vi "ActiView806-Lores.vi"() -> ()   [LabVIEW 2020] (continued)
          # "Average Cluster"
          # "Tab Control"
          # "Last Call"
          # "Stop next call"
          # "Update Avg"
          # "Average Cluster"
          # "Average Total"
          # "Noise Total"
          # "Decimation Factor"
          # "Ana Filter Reset"
          # "Ana Filter Reset"
          # "Ana Channel Selection"
          # "Charts/Graphs"
          # "Ana Channel Selection"
          # "Acquisition Error"
          # "Second Half"
          # "Aux Channel Selection"
          # "Aux Channel Selection"
          # "Aux DC Reset"
          # "Aux DC Reset"
          # "Save Index"
          # "Bip Channel Selection"
          # "Bip Channel Selection"
          # "Sample Rate"
          # "Mon Channel selection"
          # "Mon Ref Selection"
          # "Mon Channel selection"
          # "Mon Ref Selection"
          # "Bip Filter Reset"
          # "Bip Filter Reset"
          # "Mon Filter Reset"
          # "Mon Filter Reset"
          # "Max/Min Display Blocksize"
          # "Popup Change"
          # "Popups Change"
          # "Max/Min Display Blocksize"
          # "Screen Reset"
          # "Current File in Byte"
          # "Header Lenght in Byte"
          # "Header Lenght in Byte"
          # "Current File in Byte"
          # "Screen Reset"
          # "Sync Error Cluster"
          # "Sync Error Cluster"
          # "Display/Save data until an error occurs,\nor Stop or Start-File button is pressed"
          # "No Incoming Data"
          # "Buffer Pointer"
          # "Buffer pointer"
          # "Speed/Save Cluster"
          # "Start Saving"
          # "New Total Buffered"
          # "Save Array"
          # "Diplay Blocksize"
          # "Display Index"
          # "Display Blocksize"
          # "New Total Displayed"
          # "Total ADC Samples/s"
          # "New Total Buffered"
          # "Buffer Size in I32"
          # "Old Total Displayed"
          # "New Total Buffered"
          # "Display Index"
          # "Old total buffered"
          n1262 = property class="VI"() -> ("Front Panel Window:Is Frontmost"=w2860:bool)  [unwired: 2 in, 2 out]
          n1263 = global write "StopThreads.glb" "StopThreads"(w2775) -> ()
          n1264 = Wait (ms)(milliseconds to wait=u32 0) -> ()  [unwired: 1 out]
          n1265 = call-poly <vilib>:"Acquire Input Data.vi"("device ID"=w2889, "error in (no error)"=w2888) -> ("device ID"=w2884:refnum<k1>, "keys pressed"=w2864:T29, "error out"=w2885:errorcluster)  [unwired: 15 out]
          n1266 = Less Or Equal?(x=w2910, y=w2905) -> (x <= y?=w2916:bool)
          n1267 = Select(t=w2910, s=w2916, f=w2905) -> (s? t:f=w2911:i64)
          n1268 = call "AVTCP-Pause FGV.vi"() -> ("Value out"=w2757:bool)  [unwired: 7 in]
          n1269 = Greater Or Equal?(x=w2842, y="RecTimeLimit") -> (x >= y?=w2810:bool)
          n1270 = Multiply(x=w2909, y="FileLimit") -> (x*y=w2813:i64)
          n1271 = global read "TCPidentification.glb" "TCP cluster"() -> (w2829:T9)
          n1272 = Quotient & Remainder(x=w2911, y=w2904) -> (floor(x/y)=w2914:i64)  [unwired: 1 out]
          n1273 = property on="MonFree" class="LstBox (strict)"() -> ("Key Focus"=w2791:bool)  [unwired: 2 in, 2 out]
          n1274 = property on="RefFree" class="LstBox (strict)"() -> ("Key Focus"=w2790:bool)  [unwired: 2 in, 2 out]
          n1275 = property on="BipFree" class="LstBox (strict)"() -> ("Key Focus"=w2789:bool)  [unwired: 2 in, 2 out]
          n1276 = property on="AnaFree" class="LstBox (strict)"() -> ("Key Focus"=w2788:bool)  [unwired: 2 in, 2 out]
          n1277 = property on="AnaOffset" class="Ring (strict)"() -> ("Key Focus"=w2786:bool)  [unwired: 2 in, 2 out]
          n1278 = Unbundle By Name(w2875) -> ("ElecGain"=w2876:i8)
          n1279 = Bundle(w2905, w2904) -> (w2805:cluster{i64, i64})  [unwired: 1 out]
          n1280 = Unbundle By Name(w2922) -> ("Valid Sweeps"=w2785:i32, "Rejected Sweeps"=w2783:i32)
          n1281 = And(x=w2757, y="Pause Saving") -> (x .and. y?=w2756:bool)
          n1282 = Select(t=T5."Disabled and Grayed Out" ("Disabled"), s="Averaging", f=T5."Enabled" ("Disabled")) -> (s? t:f=w2779:T5)
          n1283 = Less Or Equal To 0?(x=w2914) -> (x <= 0?=w2915:bool)
          n1284 = local write "Pause Saving"(w2756) -> ()
          n1285 = Select(t=i64 1, s=w2915, f=w2914) -> (s? t:f=w2912:i64)
          n1286 = Compound Arithmetic op=OR(w2791, w2790, w2789, w2788, w2786) -> (w2787:bool)
          n1287 = Unbundle By Name(w2829) -> ("connection ID"=w2824:refnum<k5>, "remote address"=→"Remote Address":string, "remote port"=w2827:u16)
          "Receive Remote Port" <- w2827
          n1288 = Unbundle By Name(w2869) -> ("Save Subset"=w2868:i8)
          n1289 = Multiply(x=w2912, y=w2904) -> (x*y=w2892:i64)
          n1290 = local read "Valid Sweeps"() -> (w2784:i32)
          n1291 = property on="AvgTrigSel" class="LstBox (strict)"("Disabled"=w2779) -> ()  [unwired: 2 in, 2 out]
          n1292 = property on="AvgTrigLog" class="Ring (strict)"("Disabled"=w2779) -> ()  [unwired: 2 in, 2 out]
          n1293 = property on="AvgSweep" class="DigNum (strict)"("Disabled"=w2779) -> ()  [unwired: 2 in, 2 out]
          n1294 = Add(x=w2953, y=w2811) -> (x+y=w2896:i64)
          n1295 = property on="MonLPfreq" class="DigNum (strict)"() -> ("Key Focus"=w2859:bool)  [unwired: 2 in, 2 out]
          n1296 = property on="MonHPfreq" class="DigNum (strict)"() -> ("Key Focus"=w2858:bool)  [unwired: 2 in, 2 out]
          n1297 = property on="BipLPfreq" class="DigNum (strict)"() -> ("Key Focus"=w2857:bool)  [unwired: 2 in, 2 out]
          n1298 = property on="BipHPfreq" class="DigNum (strict)"() -> ("Key Focus"=w2856:bool)  [unwired: 2 in, 2 out]
          n1299 = property on="AvgSweep" class="DigNum (strict)"() -> ("Key Focus"=w2855:bool)  [unwired: 2 in, 2 out]
          n1300 = property on="AvgLPfreq" class="DigNum (strict)"() -> ("Key Focus"=w2854:bool)  [unwired: 2 in, 2 out]
          n1301 = property on="AvgHPfreq" class="DigNum (strict)"() -> ("Key Focus"=w2853:bool)  [unwired: 2 in, 2 out]
          n1302 = Equal To 0?(x=w2897) -> (x = 0?=w2895:bool)
          n1303 = Equal?(x=w2868, y=i8 8) -> (x = y?=w2866:bool)
          n1304 = local read "Charts/Graphs"() -> (w2924:T2)
          n1305 = Greater?(x=w2785, y=w2784) -> (0:w2781:bool)
          n1306 = Not Equal To 0?(x=w2827) -> (x != 0?=w2826:bool)
          "TCP Connected" <- w2826
          n1307 = local read "Rejected Sweeps"() -> (w2782:i32)
          n1308 = Not And(1:w2866, 2:w2755) -> (0:w2865:bool)
          n1309 = call "AVTCP-Saving FGV.vi"("Value in"=w2755) -> ()  [unwired: 6 in, 1 out]
          n1310 = call "Act_Pointer.vi"("First Iteration"=w2895, "Handle In"=w2766, "Display Blocksize In"=w2892, "Buffer Size"=w2893, "Old Total Displayed"=w3002, "Old Total Buffered"=w3003) -> ("Data Ready"=w2963:bool, "No Incoming Data"=w2898:bool, "Buffer Pointer"=w2764:i64, "New Total Buffered"=w2899:i64, "Handle Out"=w2765:i64)
          n1311 = Greater?(x=w2896, y=w2813) -> (0:w2809:bool)
          n1312 = property on="MonFreeAvg1" class="LstBox (strict)"("Disabled"=w2779) -> ()  [unwired: 2 in, 2 out]
          n1313 = property on="RefFreeAvg1" class="LstBox (strict)"("Disabled"=w2779) -> ()  [unwired: 2 in, 2 out]
          n1314 = Compound Arithmetic op=OR(w2787, w2859, w2858, w2857, w2856, w2855, w2854, w2853) -> (w2794:bool)
          n1315 = Greater?(x=w2783, y=w2782) -> (0:w2780:bool)
          n1316 = case shown="True" w2755 {
            tunnel: w2756 -> [_ w3024]
            frame False {
            }
            frame True {
              n1317 = property on="Start Saving" class="Bool (strict)"() -> ("Colors [4]"=w3033:cluster{u32, u32}[])  [unwired: 2 in, 2 out]
              n1318 = Select(t="Not Saving" ("f"), s=w3024, f="Saving" ("Boolean Text.Text")) -> (s? t:f=w3036:string)
              n1319 = Select(t=u32 16711680, s=w3024, f=u32 6618880) -> (s? t:f=w3028:u32)
              n1320 = Index Array(array=w3033) -> (element #1=w3027:cluster{u32, u32}, element #2=w3030:cluster{u32, u32})  [unwired: 2 in]
              n1321 = Select(t=u32 16777215, s=w3024, f=u32 0) -> (s? t:f=w3023:u32)
              n1322 = Unbundle(w3030) -> (w3029:u32)  [unwired: 1 out]
              n1323 = Bundle(w3028, w3029) -> (w3031:cluster{u32, u32})  [unwired: 1 out]
              n1324 = Build Array(w3027, w3031) -> (w3032:cluster{u32, u32}[])
              n1325 = property on="Start Saving" class="Bool (strict)"("Boolean Text.Text"=w3036, "Colors [4]"=w3032, "Boolean Text.Text Colors:Text Color"=w3023) -> ()  [unwired: 2 in, 2 out]
            }
          }
          n1326 = Not Equal?(x=w2803, y=w2767) -> (x != y?=w2925:bool)
          n1327 = Greater Or Equal?(x=w2976, y=w2812) -> (x >= y?=w2835:bool)
          n1328 = Equal?(x=w2767, y=w2924) -> (x = y?=w2777:bool)
          n1329 = Or(x=w2781, y=w2780) -> (x .or. y?=w2778:bool)
          n1330 = Exclusive Or(1:w2834, 2:w2835) -> (0:w2833:bool)
          n1331 = Or(x=w2810, y=w2809) -> (x .or. y?=w2808:bool)
          n1332 = property on="MonFreeAvg2" class="LstBox (strict)"("Disabled"=w2779) -> ()  [unwired: 2 in, 2 out]
          n1333 = property on="RefFreeAvg2" class="LstBox (strict)"("Disabled"=w2779) -> ()  [unwired: 2 in, 2 out]
          n1334 = And(x=w2778, y=w2777) -> (x .and. y?=w2776:bool)
          n1335 = And(x=w2925, y=w2777) -> (x .and. y?=w2771:bool)
          n1336 = Not And(1:w2833, 2:w2755) -> (0:w2836:bool)
          n1337 = Not And(1:w2755, 2:w2808) -> (0:w2968:bool)
          n1338 = local write "Start"(TRUE ("Start")) -> ()
          n1339 = Select(t=w3012, s=w2963, f=w3013) -> (s? t:f=w2838:i8)
          n1340 = property on="AvgScale" class="DigNum (strict)"() -> ("Key Focus"=w2852:bool)  [unwired: 2 in, 2 out]
          n1341 = property on="AvgAbsReject" class="DigNum (strict)"() -> ("Key Focus"=w2851:bool)  [unwired: 2 in, 2 out]
          n1342 = property on="AvgRelReject" class="DigNum (strict)"() -> ("Key Focus"=w2850:bool)  [unwired: 2 in, 2 out]
          n1343 = property on="AnaLPfreq" class="DigNum (strict)"() -> ("Key Focus"=w2849:bool)  [unwired: 2 in, 2 out]
          n1344 = property on="AnaHPfreq" class="DigNum (strict)"() -> ("Key Focus"=w2848:bool)  [unwired: 2 in, 2 out]
          n1345 = property on="FileLimit" class="DigNum (strict)"() -> ("Key Focus"=w2847:bool)  [unwired: 2 in, 2 out]
          n1346 = property on="RecTimeLimit" class="DigNum (strict)"() -> ("Key Focus"=w2846:bool)  [unwired: 2 in, 2 out]
          n1347 = Compound Arithmetic op=OR(w2776, w2775, w2771) -> (w2774:bool)
          n1348 = Not Or(1:w2756, 2:w2836) -> (0:→"Write":bool)
          n1349 = property on="AvgLP" class="Bool (strict)"("Disabled"=w2779) -> ()  [unwired: 2 in, 2 out]
          n1350 = property on="AvgLPfreq" class="DigNum (strict)"("Disabled"=w2779) -> ()  [unwired: 2 in, 2 out]
          n1351 = Not And(1:"Averaging", 2:w2774) -> (0:w2773:bool)
          n1352 = Select(t=w2838, s=w2773, f=w2927) -> (s? t:f=w2837:i8)
          n1353 = Select(t=w2837, s=w2836, f=w3011) -> (s? t:f=w2993:i8)
          n1354 = Compound Arithmetic op=OR(w2794, w2852, w2851, w2850, w2849, w2848, w2847, w2846) -> (w2793:bool)
          n1355 = property on="AvgHP" class="Bool (strict)"("Disabled"=w2779) -> ()  [unwired: 2 in, 2 out]
          n1356 = property on="AvgHPfreq" class="DigNum (strict)"("Disabled"=w2779) -> ()  [unwired: 2 in, 2 out]
          n1357 = Select(t=w2993, s=w2968, f=w2997) -> (s? t:f=w2839:i8)
          n1358 = Not(x=w2793) -> (.not. x?=w2792:bool)
          n1359 = And(x=w2860, y=w2792) -> (x .and. y?=w2861:bool)
          n1360 = Select(t=w2864, s=w2861, f=w2862) -> (s? t:f=w2863:T29)
          n1361 = Index Array(array=w2863) -> (element=w2872:T12)  [unwired: 1 in]
          n1362 = Equal?(x=w2872, y=T12."PRIOR (PG UP)") -> (x = y?=w2882:bool)
          n1363 = Equal?(x=w2872, y=T12."UP") -> (x = y?=w2886:bool)
          n1364 = Equal?(x=w2872, y=T12."NEXT") -> (x = y?=w2883:bool)
          n1365 = Equal?(x=w2872, y=T12."DOWN") -> (x = y?=w2887:bool)
          n1366 = Equal?(x=w2872, y=T12."RIGHT") -> (x = y?=w2822:bool)
          n1367 = Equal?(x=w2872, y=T12."LEFT") -> (x = y?=w2870:bool)
          n1368 = Or(x=w2870, y=w2822) -> (x .or. y?=w2821:bool)
          n1369 = case shown="\"Monopolar Display\"" w2803 {
            tunnel: w2887 -> [w3071 w3108 w3125 w3166 _]
            tunnel: w2886 -> [w3073 w3109 w3124 w3165 _]
            tunnel: w2883 -> [w3069 _ w3120 _ _]
            tunnel: w2882 -> [w3070 _ w3121 _ _]
            tunnel: w2881 -> [w3068 _ _ _ _]
            tunnel: w2876 -> [_ _ w3123 _ _]
            tunnel: w2874 -> [_ _ w3122 _ _]
            tunnel: w2865 -> [w3067 _ _ _ _]
            frame "Monopolar Display" {
              n1370 = Or(x=w3071, y=w3073) -> (x .or. y?=w3072:bool)
              n1371 = Or(x=w3069, y=w3070) -> (x .or. y?=w3066:bool)
              n1372 = And(x=w3066, y=w3067) -> (x .and. y?=w3065:bool)
              n1373 = case shown="True" w3072 {
                tunnel: w3071 -> [_ w3105]
                frame False {
                }
                frame True {
                  n1374 = local read "MonScale"() -> (w3100:i8)
                  n1375 = Increment(x=w3100) -> (x+1=w3107:i8)
                  n1376 = Decrement(x=w3100) -> (x-1=w3106:i8)
                  n1377 = Select(t=w3107, s=w3105, f=w3106) -> (s? t:f=w3104:i8)
                  n1378 = In Range and Coerce(upper limit=i8 15, x=w3104, lower limit=i8 0) -> (coerced(x)=w3099:i8)  [unwired: 1 out]
                  n1379 = local write "MonScale"(w3099) -> ()
                  n1380 = Wait (ms)(milliseconds to wait=u32 200) -> ()  [unwired: 1 out]
                }
              }
              n1381 = case shown="True" w3065 {
                tunnel: w3069 -> [_ w3079]
                tunnel: w3068 -> [_ w3077]
                frame False {
                }
                frame True {
                  n1382 = To Byte Integer(number=w3077) -> (8bit integer=w3076:i8[])
                  n1383 = local read "Channels"() -> (w3074:i8)
                  n1384 = Increment(x=w3074) -> (x+1=w3082:i8)
                  n1385 = Decrement(x=w3074) -> (x-1=w3081:i8)
                  n1386 = Select(t=w3082, s=w3079, f=w3081) -> (s? t:f=w3080:i8)
                  n1387 = while {
                    shift-right: [w3090] -> w3075
                    shift-left: w3080 -> [w3093]
                    tunnel: w3079 -> [w3095]
                    tunnel: w3076 -> [w3083]
                    stop <- w3084 stop-if-true
                    w3088 = i8 14 ("upper limit")
                    n1388 = Decrement(x=w3093) -> (x-1=w3096:i8)
                    n1389 = Increment(x=w3093) -> (x+1=w3097:i8)
                    n1390 = Search 1D Array(1D array=w3083, element=w3093) -> (index of element=w3098:i32)  [unwired: 1 out]
                    n1391 = Select(t=w3097, s=w3095, f=w3096) -> (s? t:f=w3094:i8)
                    n1392 = Less Than 0?(x=w3098) -> (x < 0?=w3085:bool)
                    n1393 = Select(t=w3093, s=w3085, f=w3094) -> (s? t:f=w3091:i8)
                    n1394 = Less Or Equal?(x=w3091, y=w3088) -> (x <= y?=w3087:bool)
                    n1395 = Select(t=w3091, s=w3087, f=i8 0 ("t")) -> (s? t:f=w3089:i8)
                    n1396 = Greater Or Equal To 0?(x=w3089) -> (x >= 0?=w3086:bool)
                    n1397 = Compound Arithmetic op=AND(w3086, w3087, w3085) -> (w3084:bool)
                    n1398 = Select(t=w3089, s=w3086, f=w3088) -> (s? t:f=w3090:i8)
                  }
                  n1399 = local write "Channels"(w3075) -> ()
                  n1400 = Wait (ms)(milliseconds to wait=u32 200) -> ()  [unwired: 1 out]
                }
              }
            }
            frame "Bipolar Leads" {
              n1401 = Or(x=w3108, y=w3109) -> (x .or. y?=w3110:bool)
              n1402 = case shown="True" w3110 {
                tunnel: w3108 -> [_ w3117]
                frame False {
                }
                frame True {
                  n1403 = local read "BipScale"() -> (w3111:i8)
                  n1404 = Increment(x=w3111) -> (x+1=w3119:i8)
                  n1405 = Decrement(x=w3111) -> (x-1=w3118:i8)
                  n1406 = Select(t=w3119, s=w3117, f=w3118) -> (s? t:f=w3116:i8)
                  n1407 = In Range and Coerce(upper limit=i8 15, x=w3116, lower limit=i8 0) -> (coerced(x)=w3112:i8)  [unwired: 1 out]
                  n1408 = local write "BipScale"(w3112) -> ()
                  n1409 = Wait (ms)(milliseconds to wait=u32 200) -> ()  [unwired: 1 out]
                }
              }
            }
            frame "Electrode Offset" {
              n1410 = Or(x=w3120, y=w3121) -> (x .or. y?=w3126:bool)
              n1411 = Or(x=w3125, y=w3124) -> (x .or. y?=w3127:bool)
              n1412 = case shown="True" w3127 {
                tunnel: w3125 -> [_ w3160]
                tunnel: w3123 -> [_ w3153]
                frame False {
                }
                frame True {
                  n1413 = local read "OffsetScale"() -> (w3156:i8)
                  n1414 = Increment(x=w3156) -> (x+1=w3162:i8)
                  n1415 = Decrement(x=w3156) -> (x-1=w3161:i8)
                  n1416 = Select(t=w3162, s=w3160, f=w3161) -> (s? t:f=w3159:i8)
                  n1417 = case shown="1" w3153 {
                    tunnel: [i8 3 ("upper limit") i8 4 ("upper limit")] -> w3154
                    frame 0, Default {
                    }
                    frame 1 {
                    }
                  }
                  n1418 = In Range and Coerce(upper limit=w3154, x=w3159, lower limit=i8 0) -> (coerced(x)=w3155:i8)  [unwired: 1 out]
                  n1419 = local write "OffsetScale"(w3155) -> ()
                  n1420 = Wait (ms)(milliseconds to wait=u32 200) -> ()  [unwired: 1 out]
                }
              }
              n1421 = case shown="True" w3126 {
                tunnel: w3120 -> [_ w3133]
                tunnel: w3122 -> [_ w3130]
                frame False {
                }
                frame True {
                  n1422 = To Byte Integer(number=w3130) -> (8bit integer=w3131:i8[])
                  n1423 = local read "Offset"() -> (w3128:i8)
                  n1424 = Increment(x=w3128) -> (x+1=w3136:i8)
                  n1425 = Decrement(x=w3128) -> (x-1=w3135:i8)
                  n1426 = Select(t=w3136, s=w3133, f=w3135) -> (s? t:f=w3134:i8)
                  n1427 = while {
                    shift-right: [w3144] -> w3129
                    shift-left: w3134 -> [w3147]
                    tunnel: w3133 -> [w3149]
                    tunnel: w3131 -> [w3137]
                    stop <- w3138 stop-if-true
                    w3142 = i8 4 ("upper limit")
                    n1428 = Decrement(x=w3147) -> (x-1=w3150:i8)
                    n1429 = Increment(x=w3147) -> (x+1=w3151:i8)
                    n1430 = Search 1D Array(1D array=w3137, element=w3147) -> (index of element=w3152:i32)  [unwired: 1 out]
                    n1431 = Select(t=w3151, s=w3149, f=w3150) -> (s? t:f=w3148:i8)
                    n1432 = Less Than 0?(x=w3152) -> (x < 0?=w3139:bool)
                    n1433 = Select(t=w3147, s=w3139, f=w3148) -> (s? t:f=w3145:i8)
                    n1434 = Less Or Equal?(x=w3145, y=w3142) -> (x <= y?=w3141:bool)
                    n1435 = Select(t=w3145, s=w3141, f=i8 0 ("t")) -> (s? t:f=w3143:i8)
                    n1436 = Greater Or Equal To 0?(x=w3143) -> (x >= 0?=w3140:bool)
                    n1437 = Compound Arithmetic op=AND(w3140, w3141, w3139) -> (w3138:bool)
                    n1438 = Select(t=w3143, s=w3140, f=w3142) -> (s? t:f=w3144:i8)
                  }
                  n1439 = local write "Offset"(w3129) -> ()
                  n1440 = Wait (ms)(milliseconds to wait=u32 200) -> ()  [unwired: 1 out]
                }
              }
            }
            frame "Analog Input Box" {
              n1441 = Or(x=w3166, y=w3165) -> (x .or. y?=w3167:bool)
              n1442 = case shown="True" w3167 {
                tunnel: w3166 -> [_ w3174]
                frame False {
                }
                frame True {
                  n1443 = local read "AnaScale"() -> (w3169:i8)
                  n1444 = Increment(x=w3169) -> (x+1=w3176:i8)
                  n1445 = Decrement(x=w3169) -> (x-1=w3175:i8)
                  n1446 = Select(t=w3176, s=w3174, f=w3175) -> (s? t:f=w3173:i8)
                  n1447 = In Range and Coerce(upper limit=i8 15, x=w3173, lower limit=i8 0) -> (coerced(x)=w3168:i8)  [unwired: 1 out]
                  n1448 = local write "AnaScale"(w3168) -> ()
                  n1449 = Wait (ms)(milliseconds to wait=u32 200) -> ()  [unwired: 1 out]
                }
              }
            }
            frame "About ActiView", Default {
            }
          }
          n1450 = case shown="True" w2821 {
            tunnel: w2803 -> [w3039 w3045]
            tunnel: w2822 -> [_ w3043]
            tunnel: [w3039 w3040] -> w2823
            tunnel: w2820 -> [_ w3042]
            frame False {
            }
            frame True {
              n1451 = Increment(x=w3045) -> (x+1=w3047:T2)
              n1452 = Decrement(x=w3045) -> (x-1=w3046:T2)
              n1453 = Select(t=w3047, s=w3043, f=w3046) -> (s? t:f=w3041:T2)
              n1454 = while {
                tunnel: w3043 -> [w3061]
                tunnel: w3042 -> [w3053]
                shift-right: [w3050] -> w3040
                shift-left: w3041 -> [w3051]
                stop <- w3054 stop-if-true
                w3048 = T2."About ActiView" ("Charts/Graphs")
                n1455 = To Long Integer(number=w3051) -> (32bit integer=w3052:i32)
                n1456 = Decrement(x=w3051) -> (x-1=w3062:T2)
                n1457 = Increment(x=w3051) -> (x+1=w3063:T2)
                n1458 = Search 1D Array(1D array=w3053, element=w3052) -> (index of element=w3064:i32)  [unwired: 1 out]
                n1459 = Select(t=w3063, s=w3061, f=w3062) -> (s? t:f=w3060:T2)
                n1460 = Less Than 0?(x=w3064) -> (x < 0?=w3055:bool)
                n1461 = Select(t=w3051, s=w3055, f=w3060) -> (s? t:f=w3059:T2)
                n1462 = Less Or Equal?(x=w3059, y=w3048) -> (x <= y?=w3057:bool)
                n1463 = Select(t=w3059, s=w3057, f=T2."Monopolar Display" ("Charts/Graphs")) -> (s? t:f=w3058:T2)
                n1464 = Greater Or Equal To 0?(x=w3058) -> (x >= 0?=w3056:bool)
                n1465 = Compound Arithmetic op=AND(w3056, w3057, w3055) -> (w3054:bool)
                n1466 = Select(t=w3058, s=w3056, f=w3048) -> (s? t:f=w3050:T2)
              }
              n1467 = local write "Charts/Graphs"(w3040) -> ()
              n1468 = Wait (ms)(milliseconds to wait=u32 200) -> ()  [unwired: 1 out]
            }
          }
          n1469 = property on="Trigger Chart" class="WFChart (strict)"() -> ("X Scale.Range:Maximum"=w2934:dbl)  [unwired: 2 in, 2 out]
          n1470 = property on="Mon Chart" class="WFChart (strict)"() -> ("X Scale.Range:Maximum"=w2992:dbl)  [unwired: 2 in, 2 out]
          n1471 = property on="Bip Chart" class="WFChart (strict)"() -> ("X Scale.Range:Maximum"=w2990:dbl)  [unwired: 2 in, 2 out]
          n1472 = property on="Aux Chart" class="WFChart (strict)"() -> ("X Scale.Range:Maximum"=w2973:dbl)  [unwired: 2 in, 2 out]
          n1473 = property on="Jazz Chart" class="WFChart (strict)"() -> ("XScale.Maximum"=w2801:dbl)  [unwired: 2 in, 2 out]
          n1474 = property on="Ana Chart" class="WFChart (strict)"() -> ("X Scale.Range:Maximum"=w2960:dbl)  [unwired: 2 in, 2 out]
          n1475 = case shown="1" w2839 {
            tunnel: [w3326 w3738 w4796 w4868 w4993] -> w3014
            tunnel: [w3290 w3557 w4761 w4841 w4956] -> w2900
            tunnel: w2893 -> [_ w3587 _ _ _]
            tunnel: w3002 -> [w3326 w3736 w4796 w4868 w4993]
            tunnel: w2892 -> [w3324 w3586 w4784 w4867 w4992]
            tunnel: w2899 -> [_ w3745 _ _ _]
            tunnel: [w3324 w3584 w4784 w4867 w4992] -> w2890
            tunnel: w2812 -> [_ _ w4733 w4818 _]
            tunnel: [w3302 w3662 w4792 w4834 w4960] -> w3010
            tunnel: w3009 -> [w3301 w3537 w4751 w4838 w4960]
            tunnel: [w3323 w3530 w4735 w4836 w4959] -> w3008
            tunnel: w2999 -> [w3323 w3530 w4754 w4837 w4959]
            tunnel: [w3322 w3740 w4795 w4866 w4991] -> w2991
            tunnel: w2923 -> [w3322 w3741 w4795 w4866 w4991]
            tunnel: w2756 -> [_ w3510 w4743 _ _]
            tunnel: [w3321 w3698 w4749 w4865 w4990] -> w3007
            tunnel: w2977 -> [w3321 w3458 w4749 w4865 w4990]
            tunnel: w2994 -> [_ w3737 _ _ _]
            tunnel: w2869 -> [w3303 w3512 w4778 w4856 w4979]
            tunnel: w3006 -> [_ w3448 _ _ _]
            tunnel: [w3320 w3660 w4794 w4864 w4989] -> w3005
            tunnel: w3004 -> [w3320 w3716 w4794 w4864 w4989]
            tunnel: w3001 -> [w3319 w3377 w4793 w4863 w4988]
            tunnel: [w3319 w3375 w4793 w4863 w4988] -> w3000
            tunnel: [w3291 w3454 w4756 w4835 FALSE] -> w2961
            tunnel: w2954 -> [w3317 w3744 w4768 w4822 w4986]
            tunnel: w2953 -> [w3318 w3743 w4785 w4832 w4987]
            tunnel: [w3318 w3743 w4769 w4831 w4987] -> w2996
            tunnel: [w3317 w3744 w4768 w4822 w4986] -> w2995
            tunnel: w2992 -> [_ w3666 _ _ _]
            tunnel: w2805 -> [_ w3735 _ _ _]
            tunnel: w2990 -> [_ w3667 _ _ _]
            tunnel: w2989 -> [w3316 w3609 w4783 w4862 w4985]
            tunnel: [w3316 w3707 w4783 w4862 w4985] -> w2988
            tunnel: w2986 -> [w3315 w3720 w4782 w4861 w4984]
            tunnel: [w3315 w3576 w4782 w4861 w4984] -> w2985
            tunnel: w2984 -> [_ w3416 _ _ w4963]
            tunnel: [w3314 w3572 w4781 w4860 w4983] -> w2983
            tunnel: w2982 -> [w3314 w3683 w4781 w4860 w4983]
            tunnel: w2981 -> [w3313 w3715 w4780 w4859 w4982]
            tunnel: [w3313 w3386 w4780 w4859 w4982] -> w2980
            tunnel: w2930 -> [_ w3459 _ _ _]
            tunnel: w2976 -> [w3311 w3457 w4779 w4857 w4980]
            tunnel: w2834 -> [w3312 w3714 w4747 w4858 w4981]
            tunnel: [w3311 w3699 w4779 w4857 w4980] -> w2979
            tunnel: [w3312 w3714 w4750 w4858 w4981] -> w2978
            tunnel: [w3303 w3512 w4778 w4856 w4979] -> w2761
            tunnel: w2755 -> [_ w3419 _ _ _]
            tunnel: w2975 -> [w3310 w3695 w4777 w4855 w4978]
            tunnel: [w3310 w3414 w4777 w4855 w4978] -> w2974
            tunnel: w2973 -> [_ w3668 _ _ _]
            tunnel: [w3309 w3570 w4776 w4854 w4977] -> w2971
            tunnel: w2972 -> [w3309 w3681 w4776 w4854 w4977]
            tunnel: w2970 -> [w3308 w3672 w4775 w4853 w4976]
            tunnel: [w3308 w3411 w4775 w4853 w4976] -> w2969
            tunnel: [w3284 w3668 w4730 w4815 w4950] -> w2967
            tunnel: [w3284 w3667 w4730 w4815 w4950] -> w2966
            tunnel: [w3284 w3666 w4730 w4815 w4950] -> w2965
            tunnel: [FALSE w3650 FALSE FALSE FALSE] -> w2951
            tunnel: [w3306 w3665 w4773 w4852 w4975] -> w2964
            tunnel: [w3306 w3344 w4773 w4852 w4975] -> w2907
            tunnel: w2898 -> [w3291 _ _ _ _]
            tunnel: w2960 -> [_ w3656 _ _ _]
            tunnel: [w3284 w3656 w4730 w4815 w4950] -> w2959
            tunnel: w2958 -> [w3300 w3651 w4772 w4850 w4973]
            tunnel: w2823 -> [w3299 _ w4771 w4849 _]
            tunnel: [w3300 w3410 w4772 w4850 w4973] -> w2957
            tunnel: [w3299 "Charts/Graphs" w4771 w4849 T2."Event Related Average" ("Charts/Graphs")] -> w2802
            tunnel: w2956 -> [w3298 w3568 w4770 w4848 w4972]
            tunnel: [w3298 w3571 w4770 w4848 w4972] -> w2955
            tunnel: w2950 -> [w3297 w3408 w4767 w4847 w4971]
            tunnel: w2949 -> [w3296 w3407 w4766 w4846 w4970]
            tunnel: [w3297 w3503 w4767 w4847 w4971] -> w2944
            tunnel: [w3296 w3502 w4766 w4846 w4970] -> w2945
            tunnel: w2943 -> [_ w3542 _ _ _]
            tunnel: w2940 -> [_ w3499 _ _ _]
            tunnel: [w3284 w3463 w4730 w4815 w4950] -> w2935
            tunnel: w2934 -> [_ w3463 _ _ _]
            tunnel: w2928 -> [w3294 w3637 w4764 w4844 w4947]
            tunnel: w2929 -> [w3293 w3636 w4763 w4845 w4946]
            tunnel: [w3294 w3635 w4764 w4844 w4947] -> w2933
            tunnel: [w3293 w3398 w4763 w4845 w4946] -> w2932
            tunnel: [w3295 w3633 w4765 w4843 w4940] -> w2931
            tunnel: w2922 -> [w3295 w3629 w4765 w4843 w4941]
            tunnel: "Averaging" -> [_ w3628 _ _ _]
            tunnel: w2906 -> [_ w3344 _ _ _]
            tunnel: w2819 -> [_ w3401 _ _ _]
            tunnel: w2875 -> [w3292 w3603 w4762 w4842 w4957]
            tunnel: [w3292 w3603 w4762 w4842 w4957] -> w2903
            tunnel: w2894 -> [w3290 w3588 w4761 w4841 w4956]
            tunnel: w2891 -> [_ w3585 _ _ _]
            tunnel: w2845 -> [w3289 w3561 w4760 w4840 w4955]
            tunnel: [w3289 w3560 w4760 w4840 w4955] -> w2844
            tunnel: w2842 -> [w3288 w3559 w4753 w4839 w4954]
            tunnel: [w3288 w3559 w4757 w4839 w4954] -> w2843
            tunnel: w2841 -> [w3287 w3558 w4755 w4825 w4953]
            tunnel: [w3287 w3558 w4755 w4833 w4953] -> w2840
            tunnel: w2810 -> [_ _ _ w4830 _]
            tunnel: w2813 -> [_ _ _ w4820 _]
            tunnel: w2832 -> [_ w3506 _ _ _]
            tunnel: w2831 -> [_ w3532 _ _ _]
            tunnel: w2830 -> [_ w3531 _ _ _]
            tunnel: w2826 -> [_ w3534 _ _ _]
            tunnel: w2825 -> [_ w3538 _ _ _]
            tunnel: w2824 -> [_ w3533 _ _ _]
            tunnel: w2818 -> [w3286 w3494 w4739 w4819 w4952]
            tunnel: [w3286 "Box" w4739 w4819 w4952] -> w2817
            tunnel: w2816 -> [_ w3488 _ _ _]
            tunnel: [w3285 w3465 w4737 w4816 w4951] -> w2815
            tunnel: w2807 -> [w3285 _ w4737 w4816 w4951]
            tunnel: w2806 -> [_ w3466 _ _ _]
            tunnel: [w3284 w3462 w4730 w4815 w4950] -> w2800
            tunnel: w2801 -> [_ w3462 _ _ _]
            tunnel: w2799 -> [w3282 w3442 w4728 w4813 w4948]
            tunnel: [w3282 w3424 w4728 w4813 w4948] -> w2798
            tunnel: w2797 -> [w3283 w3425 w4729 w4814 w4949]
            tunnel: [w3283 w3439 w4729 w4814 w4949] -> w2796
            tunnel: [w3281 w3350 w4727 w4812 w4934] -> w2769
            tunnel: w2768 -> [w3281 w3341 w4727 w4812 w4934]
            frame 0, Default {
              w3284 = 0.0 ("XScale.Maximum")
              w3306 = i64 0 ("Prop Screen Minimum")
              # "Wait"
              n1476 = Wait (ms)(milliseconds to wait=u32 10) -> ()  [unwired: 1 out]
              n1477 = Build Array(w3291) -> (w3305:bool[])
              n1478 = Boolean Array To Number(Boolean array=w3305) -> (number=w3304:u32)
              n1479 = call "Act_Error_Jazz.vi"("Error Code In"=w3304, "error in (no error)"=w3301) -> ("error out"=w3302:errorcluster)  [unwired: 2 out]
            }
            frame 1 {
              w3332 = T5."Disabled and Grayed Out" ("Disabled")
              w3426 = 262144.0  # 2^18
              w3607 = 1.0  # uV/div
              w3352 = TRUE  # Online?
              w3456 = FALSE  # No Error
              # "Screen Duration"
              # "RespSwitch"
              # "Jazz LoBatt"
              # "Reset Jazz Labels"
              # "JazzOn"
              # "<-- Mark2"
              # "First Call"
              # "<-- ADC Rate"
              # "<-- ADC Channels"
              # "Markers"
              # "Reset Aux Labels"
              # "Reset Aux Labels"
              # "Screen Duration"
              # "Busy Averaging"
              # "Start Averaging"
              # "Downsample Correction"
              # "Ana Filter Reset"
              # "Reset Ana Labels"
              # "Error Code"
              # "<-- Speed Mode"
              # "End of Screen"
              # "8 Aux Channels"
              # "First Call"
              # "<-- Center Traces"
              # "<-- Charts Tab"
              # "Decimation Factor"
              # "First Call"
              # "Reset Bip Labels"
              # "Reset Bip Labels"
              # "Busy Saving"
              # "Low Batt"
              # "New Epoch"
              # "Second Half"
              # "New Save Buffer"
              # "New Index"
              # "<-- First Call"
              # "Bip Filter Reset"
              # "First Call"
              # "Reset Mon Labels"
              # "Reset Mon Filter"
              # "Sample Rate"
              # "Mon Filter Reset"
              # "Screen X-axis reset"
              # "Popup Change"
              # "Screen DC Reset"
              # "Display"
              # "Status Channel"
              # "Sync Errors"
              # "Buffer Size"
              # "Display Blocksize"
              # "New Display Index"
              # "Old Total Displayed"
              n1480 = call "Act_Ring.vi"("Serial Data"=w3585, "Display Blocksize"=w3586, "Buffer Size"=w3587, "Old Display Index"=w3588) -> ("Data Block Out"=w3553:i32[], "New Display Index"=w3557:i64)
              n1481 = Unbundle By Name(w3603) -> ("Motherboard"=w3552:i8, "ElecGain"=w3348:i8, "RespSwitch"=w3347:i8, "PopupKiller"=w3380:i8, "BreathBelt"=w3346:i8)
              n1482 = Unbundle By Name(w3512) -> ("PauseOff"=w3514:i32, "PauseOn"=w3513:i32)
              n1483 = property on="Battery\nCapacitance" class="Slide (strict)"() -> ("Disabled"=w3641:u8)  [unwired: 2 in, 2 out]
              n1484 = Bundle("PauseOff"=w3514, "PauseOn"=w3513) -> (w3511:cluster{"PauseOff":i32, "PauseOn":i32})  [unwired: 1 out]
              n1485 = property on="GSR1 pos" class="Bool (strict)"() -> ("Disabled"=w3481:u8)  [unwired: 2 in, 2 out]
              n1486 = property on="GSR2 pos" class="Bool (strict)"() -> ("Disabled"=w3482:u8)  [unwired: 2 in, 2 out]
              n1487 = Equal To 0?(x=w3641) -> (x = 0?=w3671:bool)
              n1488 = Unbundle By Name(w3512) -> ("Mark2"=w3461:bool, "GSR16Hz"=w3460:bool, "Speed Mode"=w3327:i8, "ADC Rate"=w3451:i32, "ADC Channels"=w3450:i32, "Decimate Ratio"=w3449:i32, "Mon Channels"=w3388:i32, "Bip Channels"=w3415:i32, "Aux Channels"=w3427:i32, "Jazz Channels"=w3354:i32, "Ana Channels"=w3413:i32, "Save Subset"=w3523:i8, "Add Touchproofs"=w3527:bool, "Add Sensors"=w3420:bool, "Add Jazz"=w3421:bool, "Add Anas"=w3429:bool, "Save Box"=w3409:u32)
              n1489 = In Range and Coerce(upper limit=i8 13 ("y"), x=w3327, lower limit=i8 4 ("y")) -> (In Range?=w3328:bool)  [unwired: 1 out]
              n1490 = Equal?(x=w3327, y=i8 8) -> (x = y?=w3551:bool)
              n1491 = Not(x=w3328) -> (.not. x?=w3478:bool)
              n1492 = And(x=w3461, y=w3478) -> (x .and. y?=w3477:bool)
              n1493 = Unbundle By Name(w3629) -> ("Busy Averaging"=w3621:bool)
              n1494 = Equal To 0?(x=w3482) -> (x = 0?=w3473:bool)
              n1495 = Bundle("GsrScale"="GsrScale", "ErgoScale"="ErgoScale", "ErgoLP"="ErgoLP", "RespScale"="RespScale", "PletScale"="PletScale", "TempScale"="TempScale") -> (w3642:T30)  [unwired: 1 out]
              n1496 = Equal To 0?(x=w3481) -> (x = 0?=w3474:bool)
              n1497 = Array Size(array=w3672) -> (size(s)=w3676:i32)
              n1498 = Not(x=w3621) -> (.not. x?=w3634:bool)
              n1499 = Not Equal To 0?(x=w3354) -> (x != 0?=w3353:bool)
              n1500 = And(x=w3628, y=w3634) -> (x .and. y?=w3631:bool)
              n1501 = Decrement(x=w3427) -> (x-1=w3550:i32)
              n1502 = Unbundle By Name(w3512) -> ("Mon Channels"=w3541:i32, "Bip Channels"=w3540:i32, "Aux Channels"=w3539:i32, "Jazz Channels"=w3445:i32)
              n1503 = And(x=w3419, y=w3420) -> (x .and. y?=w3467:bool)
              n1504 = Select(t=T5."Disabled and Grayed Out" ("Disabled"), s=w3467, f=T5."Enabled" ("Disabled")) -> (s? t:f=w3664:T5)
              n1505 = And(x=w3419, y=w3421) -> (x .and. y?=w3403:bool)
              n1506 = And(x=w3419, y=w3429) -> (x .and. y?=w3468:bool)
              n1507 = property on="AuxFree" class="LstBox (strict)"("Disabled"=w3664) -> ()  [unwired: 2 in, 2 out]
              n1508 = Add(x=w3388, y=w3415) -> (x+y=w3381:i32)
              n1509 = Add(x=w3381, y="AuxFree") -> (x+y=w3411:i32[])
              n1510 = Array Size(array=w3411) -> (size(s)=w3604:i32)
              n1511 = Not Equal?(x=w3604, y=w3676) -> (x != y?=w3673:bool)
              n1512 = Not Equal?(x=w3411, y=w3672) -> (x != y?=w3675:bool[])
              n1513 = Or Array Elements(Boolean array=w3675) -> (logical OR=w3674:bool)
              n1514 = Bundle("Mon Channels"=w3541, "Bip Channels"=w3540, "Aux Channels"=w3539, "Jazz Channels"=w3445) -> (w3535:T31)  [unwired: 1 out]
              n1515 = call "Act_Screen.vi"("Screen Reset Interval"=w3344, "Max/Min Display Blocksize"=w3735, "Nr of Channels"=w3450, "New Total Buffered"=w3745, "Buffer Size"=w3587, "ADC samples/s"=w3737, "Old Display Blocksize"=w3586, "Old Total Displayed"=w3736) -> ("Screen Reset Parameters"=w3733:T32, "New Display Blocksize"=w3584:i64, "New Total Displayed"=w3738:i64, "Errors Out"=w3640:T33)
              n1516 = Unbundle By Name(w3640) -> ("Ring Buffer Overflow"=w3455:bool, "First Call"=w3431:bool)
              n1517 = Or(x=w3431, y=w3510) -> (x .or. y?=w3713:bool)
              n1518 = case shown="False" w3328 {
                tunnel: [w3833 w3875] -> w3379
                tunnel: [w3845 w3876] -> w3555
                tunnel: [w3842 w3884] -> w3554
                tunnel: [w3844 w3880] -> w3556
                tunnel: w3553 -> [w3843 w3873]
                tunnel: w3552 -> [_ w3874]
                tunnel: w3551 -> [_ w3871]
                tunnel: w3450 -> [w3841 w3883]
                tunnel: w3347 -> [w3839 w3882]
                tunnel: w3451 -> [w3837 w3881]
                tunnel: [w3840 w3878] -> w3496
                tunnel: w3461 -> [w3840 _]
                tunnel: "Box" -> [w3838 _]
                tunnel: w3460 -> [w3836 w3879]
                tunnel: [w3835 w3878] -> w3349
                tunnel: w3431 -> [w3834 w3877]
                tunnel: [T14 {"Jazz No Data"=FALSE, "Jazz Packet Loss"=FALSE, "Jazz Batt"=0, "Jazz Packet Loss 2"=FALSE} ("Jazz Cluster") w3868] -> w3371
                tunnel: w3353 -> [_ w3872]
                tunnel: w3327 -> [w3831 w3870]
                tunnel: w3346 -> [w3830 w3869]
                frame False {
                  n1519 = case shown="True" w3840 {
                    tunnel: [w3847 w3856] -> w3833
                    tunnel: [w3853 w3866] -> w3845
                    tunnel: [w3852 w3865] -> w3844
                    tunnel: w3843 -> [w3851 w3867]
                    tunnel: [T15 {"GSR2pos"=FALSE, "GSR1neg"=FALSE, "GSR1pos"=FALSE, "GSR2neg"=FALSE} ("Cluster") w3864] -> w3842
                    tunnel: w3841 -> [w3849 w3863]
                    tunnel: w3839 -> [_ w3862]
                    tunnel: w3838 -> [_ w3861]
                    tunnel: w3837 -> [_ w3860]
                    tunnel: [FALSE ("CM in Range") w3858] -> w3835
                    tunnel: w3836 -> [_ w3859]
                    tunnel: w3834 -> [_ w3857]
                    tunnel: w3831 -> [w3846 w3855]
                    tunnel: w3830 -> [_ w3854]
                    frame False {
                      n1520 = call "Convert_0-3.vi"("Nr of Channels"=w3849, "Speedmode"=w3846, "Serial In"=w3851) -> ("2D Chan Array"=w3852:i32[][], "Status Channnel"=w3853:i32[], "Number of Sync Errors"=w3847:i16)
                    }
                    frame True {
                      n1521 = call "Convert_Daisy.vi"("Serial In"=w3867, "GSR16Hz"=w3859, "Speedmode"=w3855, "BreathBelt"=w3854, "Box"=w3861, "RespSwitch"=w3862, "Nr of Channels"=w3863, "ADC Rate"=w3860, "First Call"=w3857) -> ("GSR in Range"=w3864:T34, "Number of Sync Errors"=w3856:i16, "Status Channnel"=w3866:i32[], "576 or 544 Chan Array"=w3865:i32[][], "CM in Range"=w3858:bool)  [unwired: 2 out]
                    }
                  }
                }
                frame True {
                  w3878 = FALSE
                  n1522 = call "Convert_4-8_New.vi"("Serial In"=w3873, "Jazz On"=w3872, "GSR16Hz"=w3879, "Speedmode"=w3870, "Motherboard"=w3874, "RespSwitch"=w3882, "Nr of Channels"=w3883, "ADC Rate"=w3881, "AIB"=w3871, "First Call"=w3877, "BreathBelt"=w3869) -> ("GSR in Range"=w3884:T34, "Number of Sync Errors"=w3875:i16, "Jazz Cluster"=w3868:T35, "Status Channnel"=w3876:i32[], "2D Chan Array"=w3880:i32[][])
                }
              }
              n1523 = Unbundle(w3554) -> ("GSR1pos"=w3469:bool, "GSR1neg"=w3470:bool, "GSR2pos"=w3471:bool, "GSR2neg"=w3472:bool)
              n1524 = And(x=w3474, y=w3469) -> (x .and. y?=→"GSR1 pos":bool)
              n1525 = And(x=w3474, y=w3470) -> (x .and. y?=→"GSR1 neg":bool)
              n1526 = And(x=w3473, y=w3471) -> (x .and. y?=→"GSR2 pos":bool)
              n1527 = And(x=w3473, y=w3472) -> (x .and. y?=→"GSR2 neg":bool)
              n1528 = call "Downsample.vi"("Status Channel  In"=w3555, "Online?"=w3352, "N Channel Array In"=w3556, "Start Epoch"=w3713, "Marker Cluster"=w3561, "First Call"=w3431, "Decimate Ratio"=w3449) -> ("N-1 Channel Array Out"=w3412:i32[][], "Status Channel Out"=w3406:i32[])
              n1529 = call "TrigProcess.vi"("PopupKiller"=w3380, "Pause Cluster"=w3511, "First Call"=w3431, "Pause Saving"=w3510, "Decimation Factor"=w3401, "Status Channel  In"=w3406, "Nr of Displayed Triggers"=w3506) -> ("Pause"=w3509:bool, "Lamps Cluster"=w3508:cluster{"CM in Range":bool, "Low Batt":bool}, "Triggers Boolean"=w3351:bool[][], "Triggers Chart Signals"=→"Trigger Chart":i32[][])
              n1530 = Exclusive Or(1:w3510, 2:w3509) -> (0:w3566:bool)
              n1531 = case shown="True" w3566 {
                tunnel: w3509 -> [_ w3895]
                frame False {
                }
                frame True {
                  n1532 = local write "Pause Saving"(w3895) -> ()
                }
              }
              n1533 = Unbundle By Name(w3508) -> ("CM in Range"=w3480:bool, "Low Batt"=w3507:bool)
              n1534 = Select(t=w3349, s=w3477, f=w3480) -> (s? t:f=→"CM in Range":bool)
              n1535 = Compound Arithmetic op=OR(w3431, w3674, w3673) -> (w3591:bool)
              n1536 = case shown="True" w3591 {
                tunnel: "AuxFree" -> [_ w4101]
                tunnel: w3604 -> [_ w4097]
                tunnel: w3448 -> [_ w4092]
                tunnel: w3411 -> [_ w4094]
                frame False {
                }
                frame True {
                  w4095 = 7  # Nr of Aux Labels
                  w4103 = -292.0  # Upper Y-value
                  w4105 = 532.0  # Lower Y-value
                  n1537 = Not Equal To 0?(x=w4097) -> (x != 0?=w4098:bool)
                  n1538 = Increment(x=w4097) -> (x+1=w4099:i32)
                  n1539 = stacked-sequence {
                    tunnel: w4101 -> [w4116 w4127 w4137 w4145 w4151]
                    frame #0 {
                      w4107 = T5."Disabled and Grayed Out" ("Disabled")
                      w4108 = T5."Enabled" ("Disabled")
                      w4113 = -1 ("y")
                      n1540 = Search 1D Array(1D array=w4116, element=0) -> (index of element=w4120:i32)  [unwired: 1 out]
                      n1541 = Search 1D Array(1D array=w4116, element=1) -> (index of element=w4119:i32)  [unwired: 1 out]
                      n1542 = Not Equal?(x=w4120, y=w4113) -> (x != y?=w4118:bool)
                      n1543 = Not Equal?(x=w4119, y=w4113) -> (x != y?=w4112:bool)
                      n1544 = Or(x=w4118, y=w4112) -> (x .or. y?=w4117:bool)
                      n1545 = Select(t=w4108, s=w4112, f=w4107) -> (s? t:f=w4109:T5)
                      n1546 = Select(t=w4108, s=w4118, f=w4107) -> (s? t:f=w4111:T5)
                      n1547 = Select(t=w4108, s=w4117, f=w4107) -> (s? t:f=w4110:T5)
                      n1548 = property on="GSR1 pos" class="Bool (strict)"("Disabled"=w4111) -> ()  [unwired: 2 in, 2 out]
                      n1549 = property on="GSR1 neg" class="Bool (strict)"("Disabled"=w4111) -> ()  [unwired: 2 in, 2 out]
                      n1550 = property on="GSR1" class="DigNum (strict)"("Disabled"=w4111) -> ()  [unwired: 2 in, 2 out]
                      n1551 = property on="GSR2 pos" class="Bool (strict)"("Disabled"=w4109) -> ()  [unwired: 2 in, 2 out]
                      n1552 = property on="GSR2 neg" class="Bool (strict)"("Disabled"=w4109) -> ()  [unwired: 2 in, 2 out]
                      n1553 = property on="GSR2" class="DigNum (strict)"("Disabled"=w4109) -> ()  [unwired: 2 in, 2 out]
                      n1554 = property on="GsrScale" class="Ring (strict)"("Disabled"=w4110) -> ()  [unwired: 2 in, 2 out]
                      n1555 = property on="GSR units" class="Str"("Disabled"=w4110) -> ()  [unwired: 2 in, 2 out]
                    }
                    frame #1 {
                      w4123 = -1 ("y")
                      n1556 = Search 1D Array(1D array=w4127, element=2) -> (index of element=w4132:i32)  [unwired: 1 out]
                      n1557 = Search 1D Array(1D array=w4127, element=3) -> (index of element=w4131:i32)  [unwired: 1 out]
                      n1558 = Not Equal?(x=w4132, y=w4123) -> (x != y?=w4130:bool)
                      n1559 = Not Equal?(x=w4131, y=w4123) -> (x != y?=w4129:bool)
                      n1560 = Or(x=w4130, y=w4129) -> (x .or. y?=w4128:bool)
                      n1561 = Select(t=T5."Enabled" ("Disabled"), s=w4128, f=T5."Disabled and Grayed Out" ("Disabled")) -> (s? t:f=w4124:T5)
                      n1562 = property on="ErgoScale" class="Ring (strict)"("Disabled"=w4124) -> ()  [unwired: 2 in, 2 out]
                    }
                    frame #2 {
                      n1563 = Search 1D Array(1D array=w4137, element=4) -> (index of element=w4139:i32)  [unwired: 1 out]
                      n1564 = Not Equal?(x=w4139, y=-1) -> (x != y?=w4134:bool)
                      n1565 = Select(t=T5."Enabled" ("Disabled"), s=w4134, f=T5."Disabled and Grayed Out" ("Disabled")) -> (s? t:f=w4136:T5)
                      n1566 = property on="RespScale" class="Ring (strict)"("Disabled"=w4136) -> ()  [unwired: 2 in, 2 out]
                    }
                    frame #3 {
                      n1567 = Search 1D Array(1D array=w4145, element=5) -> (index of element=w4148:i32)  [unwired: 1 out]
                      n1568 = Not Equal?(x=w4148, y=-1) -> (x != y?=w4144:bool)
                      n1569 = Select(t=T5."Enabled" ("Disabled"), s=w4144, f=T5."Disabled and Grayed Out" ("Disabled")) -> (s? t:f=w4143:T5)
                      n1570 = property on="PletScale" class="Ring (strict)"("Disabled"=w4143) -> ()  [unwired: 2 in, 2 out]
                    }
                    frame #4 {
                      n1571 = Search 1D Array(1D array=w4151, element=6) -> (index of element=w4156:i32)  [unwired: 1 out]
                      n1572 = Not Equal?(x=w4156, y=-1) -> (x != y?=w4153:bool)
                      n1573 = Select(t=T5."Enabled" ("Disabled"), s=w4153, f=T5."Disabled and Grayed Out" ("Disabled")) -> (s? t:f=w4152:T5)
                      n1574 = property on="TempScale" class="Ring (strict)"("Disabled"=w4152) -> ()  [unwired: 2 in, 2 out]
                      n1575 = property on="Degrees Celcius" class="DigNum (strict)"("Disabled"=w4152) -> ()  [unwired: 2 in, 2 out]
                    }
                  }
                  n1576 = Subtract(x=w4105, y=w4103) -> (x-y=w4104:dbl)
                  n1577 = Select(t=w4099, s=w4098, f=2) -> (s? t:f=w4093:i32)
                  n1578 = To Double Precision Float(number=w4093) -> (double precision float=w4096:dbl)
                  n1579 = Divide(x=w4104, y=w4096) -> (x/y=w4102:dbl)
                  n1580 = for {
                    N: w4095 -> [_]
                    tunnel: w4092 -> [w4164]
                    tunnel: w4094 -> [w4161]
                    tunnel: w4103 -> [w4166]
                    tunnel: w4102 -> [w4165]
                    tunnel: w4097 -> [w4162]
                    i -> [w4157]
                    n1581 = Greater?(x=w4162, y=w4157) -> (0:w4163:bool)
                    n1582 = Increment(x=w4157) -> (x+1=w4160:i32)
                    n1583 = case shown="True" w4163 {
                      tunnel: w4166 -> [_ w4194]
                      tunnel: w4165 -> [_ w4193]
                      tunnel: w4164 -> [_ w4184]
                      tunnel: w4160 -> [_ w4189]
                      tunnel: ["" w4185] -> w4159
                      tunnel: [0 w4188] -> w4158
                      tunnel: w4161 -> [_ w4187]
                      tunnel: w4157 -> [_ w4186]
                      frame False {
                      }
                      frame True {
                        n1584 = Index Array(array=w4187, index=w4186) -> (element=w4183:i32)
                        n1585 = To Double Precision Float(number=w4189) -> (double precision float=w4192:dbl)
                        n1586 = Index Array(array=w4184, index=w4183) -> (element=w4190:string)
                        n1587 = Multiply(x=w4193, y=w4192) -> (x*y=w4195:dbl)
                        n1588 = Add(x=w4194, y=w4195) -> (x+y=w4196:dbl)
                        n1589 = String Subset(string=w4190, length (rest)=4 ("length (rest)")) -> (substring=w4185:string)  [unwired: 1 out]
                        n1590 = To Long Integer(number=w4196) -> (32bit integer=w4188:i32)
                      }
                    }
                    n1591 = case shown="7, Default" w4160 {
                      tunnel: w4159 -> [w4167 w4169 w4171 w4173 w4175 w4177 w4179]
                      tunnel: w4158 -> [w4168 w4170 w4172 w4174 w4176 w4178 w4180]
                      frame 1 {
                        n1592 = property on="Aux1" class="Str"("Position:Top"=w4168) -> ()  [unwired: 2 in, 2 out]
                        "Aux1" <- w4167
                      }
                      frame 2 {
                        n1593 = property on="Aux2" class="Str"("Position:Top"=w4170) -> ()  [unwired: 2 in, 2 out]
                        "Aux2" <- w4169
                      }
                      frame 3 {
                        n1594 = property on="Aux3" class="Str"("Position:Top"=w4172) -> ()  [unwired: 2 in, 2 out]
                        "Aux3" <- w4171
                      }
                      frame 4 {
                        n1595 = property on="Aux4" class="Str"("Position:Top"=w4174) -> ()  [unwired: 2 in, 2 out]
                        "Aux4" <- w4173
                      }
                      frame 5 {
                        n1596 = property on="Aux5" class="Str"("Position:Top"=w4176) -> ()  [unwired: 2 in, 2 out]
                        "Aux5" <- w4175
                      }
                      frame 6 {
                        n1597 = property on="Aux6" class="Str"("Position:Top"=w4178) -> ()  [unwired: 2 in, 2 out]
                        "Aux6" <- w4177
                      }
                      frame 7, Default {
                        n1598 = property on="Aux7" class="Str"("Position:Top"=w4180) -> ()  [unwired: 2 in, 2 out]
                        "Aux7" <- w4179
                      }
                    }
                  }
                  n1599 = To Double Precision Float(number=w4093) -> (double precision float=w4106:dbl)
                  n1600 = property on="Aux Chart" class="WFChart (strict)"("YScale.Maximum"=w4106) -> ()  [unwired: 2 in, 2 out]
                }
              }
              n1601 = Unbundle By Name(w3371) -> ("Jazz No Data"=w3356:bool, "Jazz Packet Loss"=w3355:bool, "Jazz Batt"=w3357:u8, "Jazz New Firmware"=→"Jazz New\nFirmware":bool)
              "Jazz Batt Cap" <- w3357
              n1602 = Add(x=w3381, y=w3427) -> (x+y=w3417:i32)
              n1603 = case shown="True" w3496 {
                tunnel: w3417 -> [_ w3828]
                tunnel: w3412 -> [w3824 w3827]
                tunnel: [w3824 w3826] -> w3405
                tunnel: "Box" -> [_ w3825]
                frame False {
                }
                frame True {
                  n1604 = Multiply(x=w3825, y=w3828) -> (x*y=w3829:i32)
                  n1605 = Array Subset(array=w3827, index (row)=w3829, length (row)=w3828) -> (w3826:i32[][])  [unwired: 2 in]
                }
              }
              n1606 = Array Subset(array=w3405, index (row)=w3381, length (row)=w3427) -> (w3677:i32[][])  [unwired: 2 in]
              n1607 = call "TCP-Jazz.vi"("Status Channel  In"=w3406, "connection ID"=w3533, "TCP Connected"=w3534, "TCP Add Cluster"=w3538, "Chan Number Cluster"=w3535, "error in (no error)"=w3537, "TCP Samples/Chan"=w3531, "TCP total Bytes"=w3532, "N Channel Array In"=w3405) -> ("error out"=w3536:errorcluster, "Bytes Received by Client"=→"Bytes received by Client":i32, "Bytes Sent by Server"=→"Bytes sent by Server":i32)
              n1608 = Format Into String(format string="%d", w3357) -> (resulting string=w3370:string)  [unwired: 2 in, 1 out]
              n1609 = Equal?(x=w3523, y=i8 8) -> (x = y?=w3522:bool)
              n1610 = case shown="\"Electrode Offset\"" "Charts/Graphs" {
                tunnel: w3405 -> [w4217 _]
                tunnel: w3388 -> [w4200 _]
                tunnel: w3327 -> [w4199 _]
                tunnel: w3348 -> [w4213 _]
                tunnel: w3448 -> [w4197 _]
                tunnel: w3461 -> [w4201 _]
                frame "Electrode Offset" {
                  w4219 = 64  # Nr of Offset Labels
                  n1611 = case shown="0, Default" w4213 {
                    tunnel: [i8 3 ("x") i8 4 ("x")] -> w4224
                    frame 0, Default {
                    }
                    frame 1 {
                    }
                  }
                  n1612 = Equal?(x="OffsetScale", y=w4224) -> (x = y?=w4228:bool)
                  "Full Range" <- w4228
                  n1613 = case shown="0" "OffsetScale" {
                    tunnel: [20.0 50.0 100.0 262.0 1049.0] -> w4205
                    tunnel: [-195 ("Position:Left") -195 ("Position:Left") -200 ("Position:Left") -200 ("Position:Left") -205 ("Position:Left")] -> w4229
                    frame 0 {
                    }
                    frame 1 {
                    }
                    frame 2 {
                    }
                    frame 3, Default {
                    }
                    frame 4 {
                    }
                  }
